vi "Fase 5_Grupo 1.vi"() -> ()   [LabVIEW 2020]
panel:
  out "CantidadChoco":dbl
  out "Bool 5":bool
  out "Bool 4":bool
  out "Bool 2":bool
  out "Bool":bool
  out "ChocoBoolean":bool
  in  "BandaSlide":dbl(slide) scale=0.0..50.0
  out "Bool 3":bool
  out "CajaBool":bool
  out "ABORTAR":bool
  out "Parada":bool
  out "Marcha":bool
  in  "Abortar 4":bool
  in  "Parada 4":bool
  in  "Marcha 4":bool
  out "Fin":bool
  # "Dídier Javier Ramírez Henao"
  # "Empaquetado"
  # "Refinado"
  # "Almacenado"
  # "Subproceso 4 _ Distribución"
  # "Fin"
  # "Pulsadores de mando"
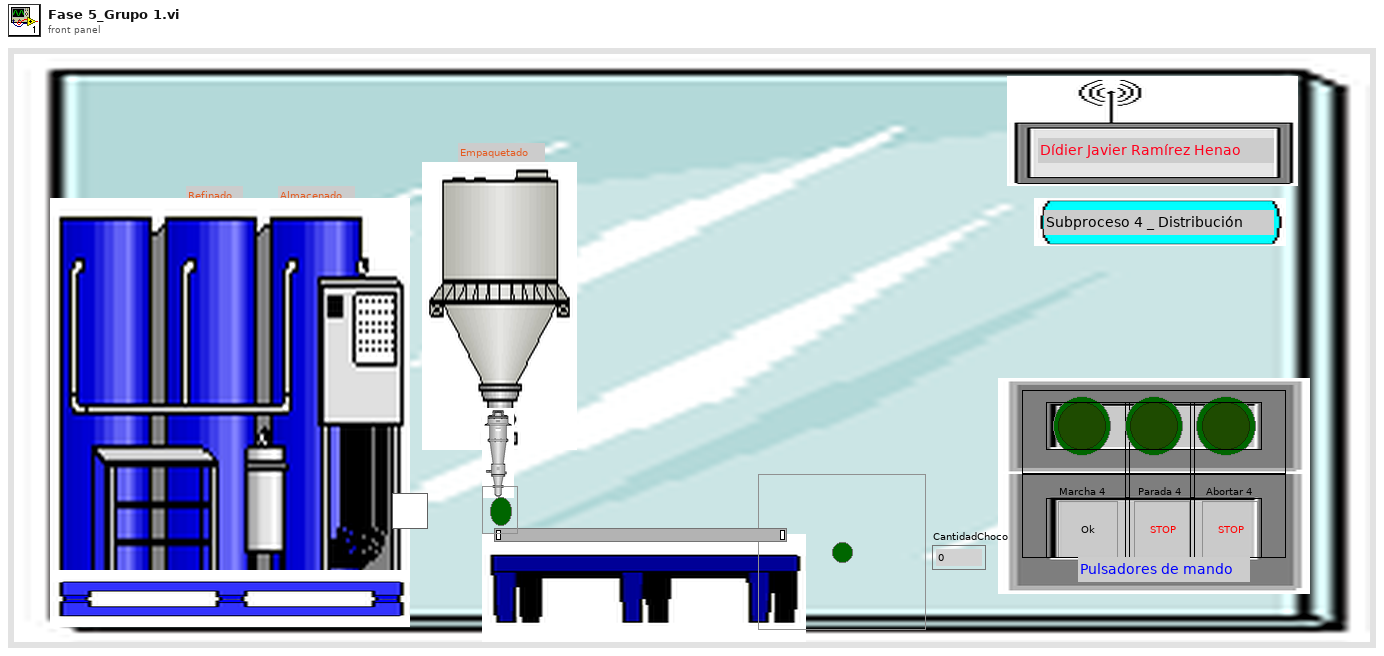
[diagram p1: front panel]
types:
  T1 = enum16{"INICIO", "MARCHA", "PARO", "ABORTAR", "FIN"}
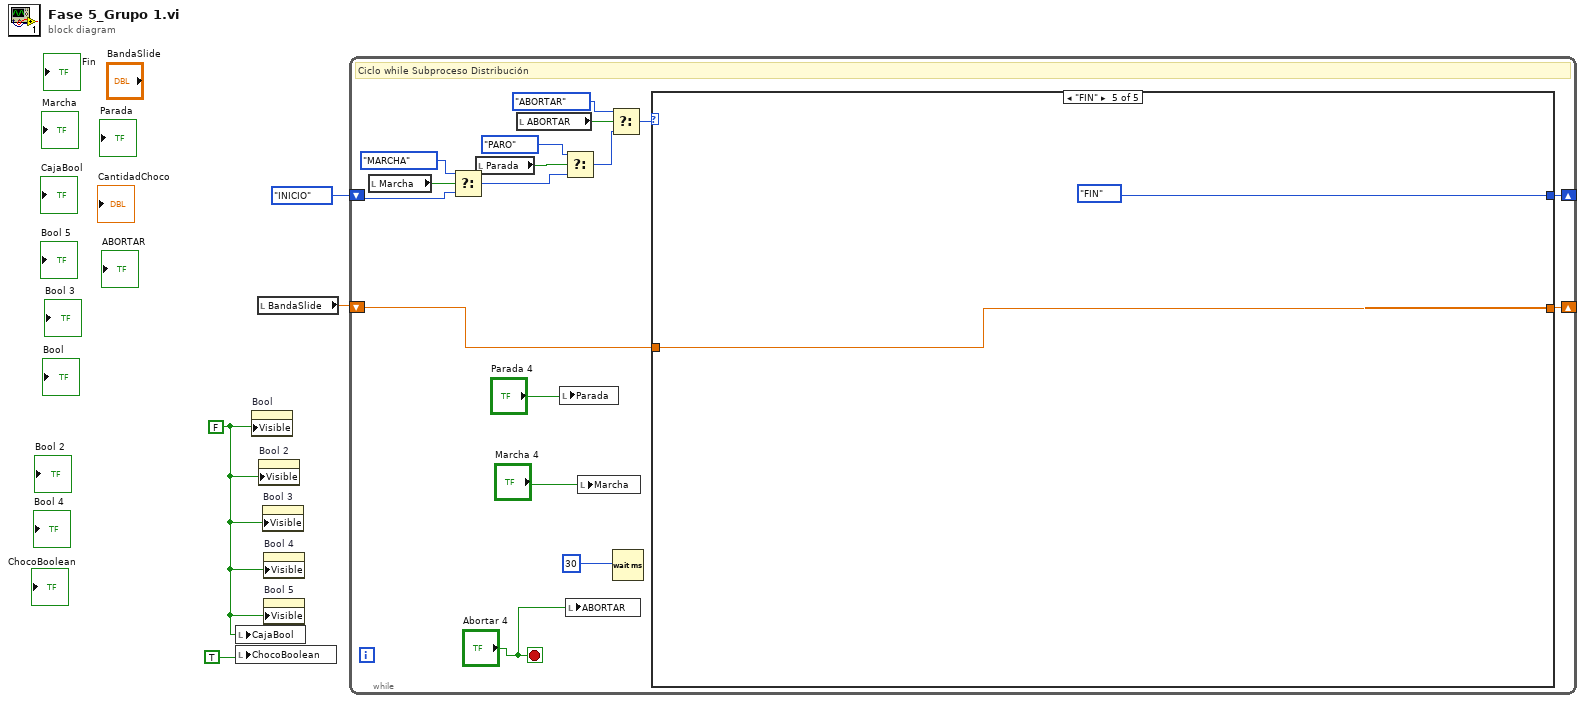
[diagram p0: block diagram]
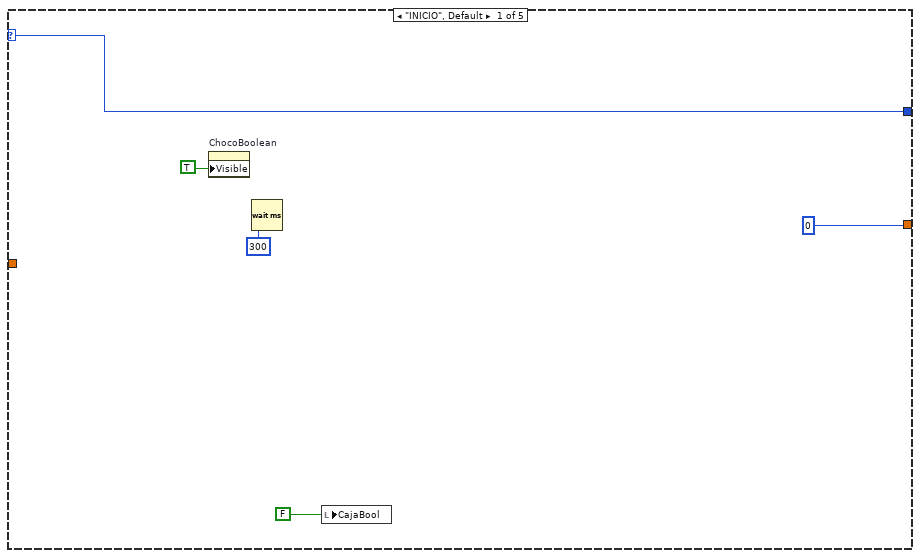
[diagram p2: hidden frame]
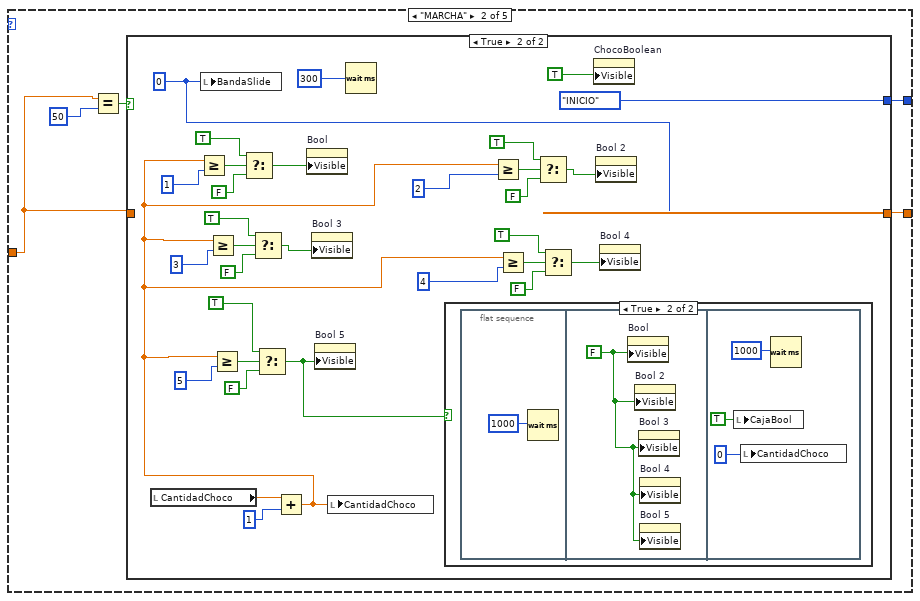
[diagram p3: hidden frame]
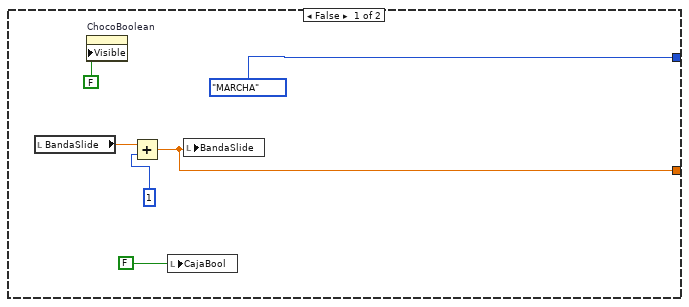
[diagram p4: hidden frame]
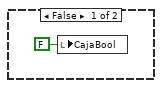
[diagram p5: hidden frame]
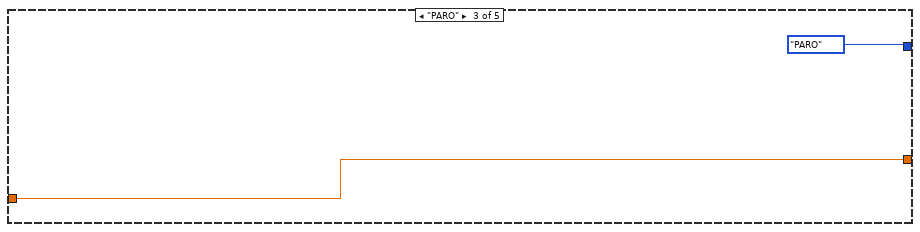
[diagram p6: hidden frame]
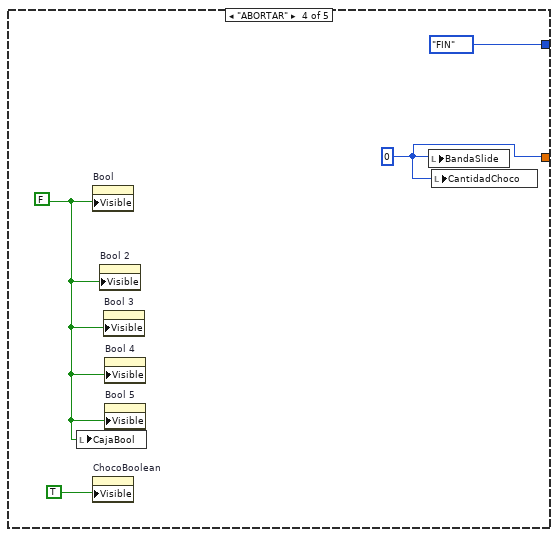
[diagram p7: hidden frame]
diagram:
  w2 = FALSE
  n1 = local write "CajaBool"(w2) -> ()
  n2 = local write "ChocoBoolean"(TRUE) -> ()
  n3 = property on="Bool" class="Bool (strict)"("Visible"=w2) -> ()  [unwired: 2 in, 2 out]
  n4 = local read "BandaSlide"() -> (w3:dbl)
  n5 = property on="Bool 2" class="Bool (strict)"("Visible"=w2) -> ()  [unwired: 2 in, 2 out]
  n6 = property on="Bool 3" class="Bool (strict)"("Visible"=w2) -> ()  [unwired: 2 in, 2 out]
  n7 = property on="Bool 4" class="Bool (strict)"("Visible"=w2) -> ()  [unwired: 2 in, 2 out]
  n8 = property on="Bool 5" class="Bool (strict)"("Visible"=w2) -> ()  [unwired: 2 in, 2 out]
  n9 = while {
    shift-right: [w8] -> _
    shift-left: T1."INICIO" -> [w19]
    shift-right: [w9] -> _
    shift-left: w3 -> [w10]
    stop <- "Abortar 4" stop-if-true
    # "Ciclo while Subproceso Distribución"
    n10 = local read "Marcha"() -> (w20:bool)
    n11 = Select(t=T1."MARCHA", s=w20, f=w19) -> (s? t:f=w17:T1)
    n12 = local read "Parada"() -> (w18:bool)
    n13 = local read "ABORTAR"() -> (w14:bool)
    n14 = local write "Parada"("Parada 4") -> ()
    n15 = Select(t=T1."PARO", s=w18, f=w17) -> (s? t:f=w12:T1)
    n16 = local write "ABORTAR"("Abortar 4") -> ()
    n17 = local write "Marcha"("Marcha 4") -> ()
    n18 = Select(t=T1."ABORTAR", s=w14, f=w12) -> (s? t:f=w11:T1)
    n19 = Wait (ms)(milliseconds to wait=30) -> ()  [unwired: 1 out]
    n20 = case shown="\"FIN\"" w11 {
      selector: w11 -> [w26 _ _ _ _]
      tunnel: w10 -> [_ w27 w77 _ w82]
      tunnel: [0 w28 w77 w80 w82] -> w9
      tunnel: [w26 w29 T1."PARO" T1."FIN" T1."FIN"] -> w8
      frame "INICIO", Default {
        n21 = property on="ChocoBoolean" class="Bool (strict)"("Visible"=TRUE) -> ()  [unwired: 2 in, 2 out]
        n22 = Wait (ms)(milliseconds to wait=300) -> ()  [unwired: 1 out]
        n23 = local write "CajaBool"(FALSE) -> ()
      }
      frame "MARCHA" {
        n24 = Equal?(x=w27, y=50) -> (x = y?=w30:bool)
        n25 = case shown="True" w30 {
          tunnel: [T1."MARCHA" T1."INICIO"] -> w29
          tunnel: [w34 w59] -> w28
          tunnel: w27 -> [_ _]
          frame False {
            n26 = local read "BandaSlide"() -> (w36:dbl)
            n27 = property on="ChocoBoolean" class="Bool (strict)"("Visible"=FALSE) -> ()  [unwired: 2 in, 2 out]
            n28 = Add(x=w36, y=1) -> (x+y=w34:dbl)
            n29 = local write "CajaBool"(FALSE) -> ()
            n30 = local write "BandaSlide"(w34) -> ()
          }
          frame True {
            w59 = 0
            n31 = local read "CantidadChoco"() -> (w66:dbl)
            n32 = local write "BandaSlide"(w59) -> ()
            n33 = Add(x=w66, y=1) -> (x+y=w39:dbl)
            n34 = Greater Or Equal?(x=w39, y=1) -> (x >= y?=w64:bool)
            n35 = Greater Or Equal?(x=w39, y=3) -> (x >= y?=w51:bool)
            n36 = Greater Or Equal?(x=w39, y=5) -> (x >= y?=w49:bool)
            n37 = Select(t=TRUE, s=w64, f=FALSE) -> (s? t:f=w60:bool)
            n38 = Select(t=TRUE, s=w51, f=FALSE) -> (s? t:f=w50:bool)
            n39 = Select(t=TRUE, s=w49, f=FALSE) -> (s? t:f=w38:bool)
            n40 = property on="Bool" class="Bool (strict)"("Visible"=w60) -> ()  [unwired: 2 in, 2 out]
            n41 = property on="Bool 3" class="Bool (strict)"("Visible"=w50) -> ()  [unwired: 2 in, 2 out]
            n42 = property on="Bool 5" class="Bool (strict)"("Visible"=w38) -> ()  [unwired: 2 in, 2 out]
            n43 = local write "CantidadChoco"(w39) -> ()
            n44 = Wait (ms)(milliseconds to wait=300) -> ()  [unwired: 1 out]
            n45 = case shown="True" w38 {
              frame False {
                n46 = local write "CajaBool"(FALSE) -> ()
              }
              frame True {
                n47 = flat-sequence {
                  frame #0 {
                    n48 = Wait (ms)(milliseconds to wait=1000) -> ()  [unwired: 1 out]
                  }
                  frame #1 {
                    w72 = FALSE
                    n49 = property on="Bool" class="Bool (strict)"("Visible"=w72) -> ()  [unwired: 2 in, 2 out]
                    n50 = property on="Bool 2" class="Bool (strict)"("Visible"=w72) -> ()  [unwired: 2 in, 2 out]
                    n51 = property on="Bool 3" class="Bool (strict)"("Visible"=w72) -> ()  [unwired: 2 in, 2 out]
                    n52 = property on="Bool 4" class="Bool (strict)"("Visible"=w72) -> ()  [unwired: 2 in, 2 out]
                    n53 = property on="Bool 5" class="Bool (strict)"("Visible"=w72) -> ()  [unwired: 2 in, 2 out]
                  }
                  frame #2 {
                    n54 = local write "CajaBool"(TRUE) -> ()
                    n55 = local write "CantidadChoco"(0) -> ()
                    n56 = Wait (ms)(milliseconds to wait=1000) -> ()  [unwired: 1 out]
                  }
                }
              }
            }
            n57 = Greater Or Equal?(x=w39, y=2) -> (x >= y?=w55:bool)
            n58 = Greater Or Equal?(x=w39, y=4) -> (x >= y?=w44:bool)
            n59 = Select(t=TRUE, s=w55, f=FALSE) -> (s? t:f=w45:bool)
            n60 = Select(t=TRUE, s=w44, f=FALSE) -> (s? t:f=w40:bool)
            n61 = property on="ChocoBoolean" class="Bool (strict)"("Visible"=TRUE) -> ()  [unwired: 2 in, 2 out]
            n62 = property on="Bool 2" class="Bool (strict)"("Visible"=w45) -> ()  [unwired: 2 in, 2 out]
            n63 = property on="Bool 4" class="Bool (strict)"("Visible"=w40) -> ()  [unwired: 2 in, 2 out]
          }
        }
      }
      frame "PARO" {
      }
      frame "ABORTAR" {
        w80 = 0
        w79 = FALSE
        n64 = local write "CajaBool"(w79) -> ()
        n65 = property on="Bool" class="Bool (strict)"("Visible"=w79) -> ()  [unwired: 2 in, 2 out]
        n66 = property on="ChocoBoolean" class="Bool (strict)"("Visible"=TRUE) -> ()  [unwired: 2 in, 2 out]
        n67 = property on="Bool 2" class="Bool (strict)"("Visible"=w79) -> ()  [unwired: 2 in, 2 out]
        n68 = property on="Bool 3" class="Bool (strict)"("Visible"=w79) -> ()  [unwired: 2 in, 2 out]
        n69 = property on="Bool 4" class="Bool (strict)"("Visible"=w79) -> ()  [unwired: 2 in, 2 out]
        n70 = property on="Bool 5" class="Bool (strict)"("Visible"=w79) -> ()  [unwired: 2 in, 2 out]
        n71 = local write "BandaSlide"(w80) -> ()
        n72 = local write "CantidadChoco"(w80) -> ()
      }
      frame "FIN" {
      }
    }
  }
